vi "nominal asset attach dataset add tag.vi"(8 "error in (no error)":errorcluster, 9 "value":string, 10 "key":string, 11 "staging":i32) -> (0 "error out":errorcluster, 3 "function return":i32)   [LabVIEW 2020, in "client.lvlib"]
doc: "int32_t nominal_asset_attach_dataset_add_tag(int32_t staging, const char *key, const char *value);"
uses:
  client.lvlib
  bin/nominalClient_64.dll
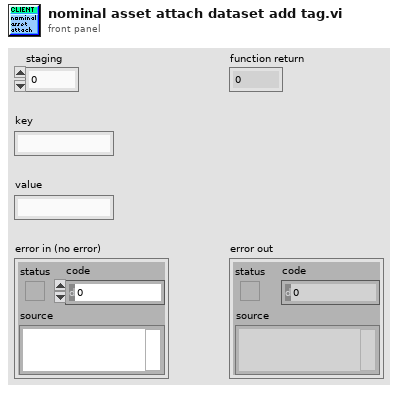
[diagram p1: front panel]
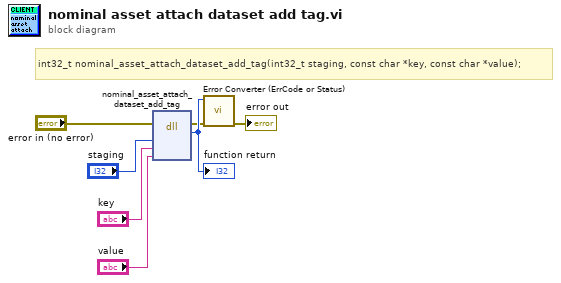
[diagram p0: block diagram]
diagram:
  # "int32_t nominal_asset_attach_dataset_add_tag(int32_t staging, const char *key, const char *value);"
  n1 = dll-call lib="C:/code/labview-client-rs/lv_src/bin/nominalClient_*.*" fn="nominal_asset_attach_dataset_add_tag"(error in="error in (no error)", "staging"="staging", "key"="key", "value"="value") -> (error out=w2:errorcluster, w7:i32)  [unwired: 5 in, 1 out]
  "function return" <- w7
  n2 = call "Error Converter (ErrCode or Status).vi"("error in (no error)"=w2, "error code"=w7) -> ("error out"=→"error out":errorcluster)  [unwired: 9 in]
